vi "Machine job id Read.vi"(11 "Machin ID":string="YSD") -> (0 "error out":errorcluster)   [LabVIEW 2015]
uses:
  Machine id selection.ctl
  PartSetup/Control 1.ctl
  <vilib>/addons/database/NI_Database_API.lvlib
  <vilib>/addons/database/Connection.llb/DB Tools Open Connec (String).vi
  <vilib>/addons/database/_DB Variant To Data/Database Variant To Data.xnode
  Galobal variable_TI.vi
panel:
  out "error out 2":errorcluster
  out "appended array":string[](array[string])
  out "Array 3":string[][](array[string])
  out "element":cluster{"Array":string[][]}
  out "data":string[][](array[string])
  out "Array 2":T1[](array[typedef])
  in  "Enum":T2
  out "Array":cluster{"Array":string[][]}[](array[cluster])
  in  "Cluster":cluster{"Array":string[][]}
  # "First motor testing Parameter"
  # "Printing Info"
  # "Second motor testing Parameter"
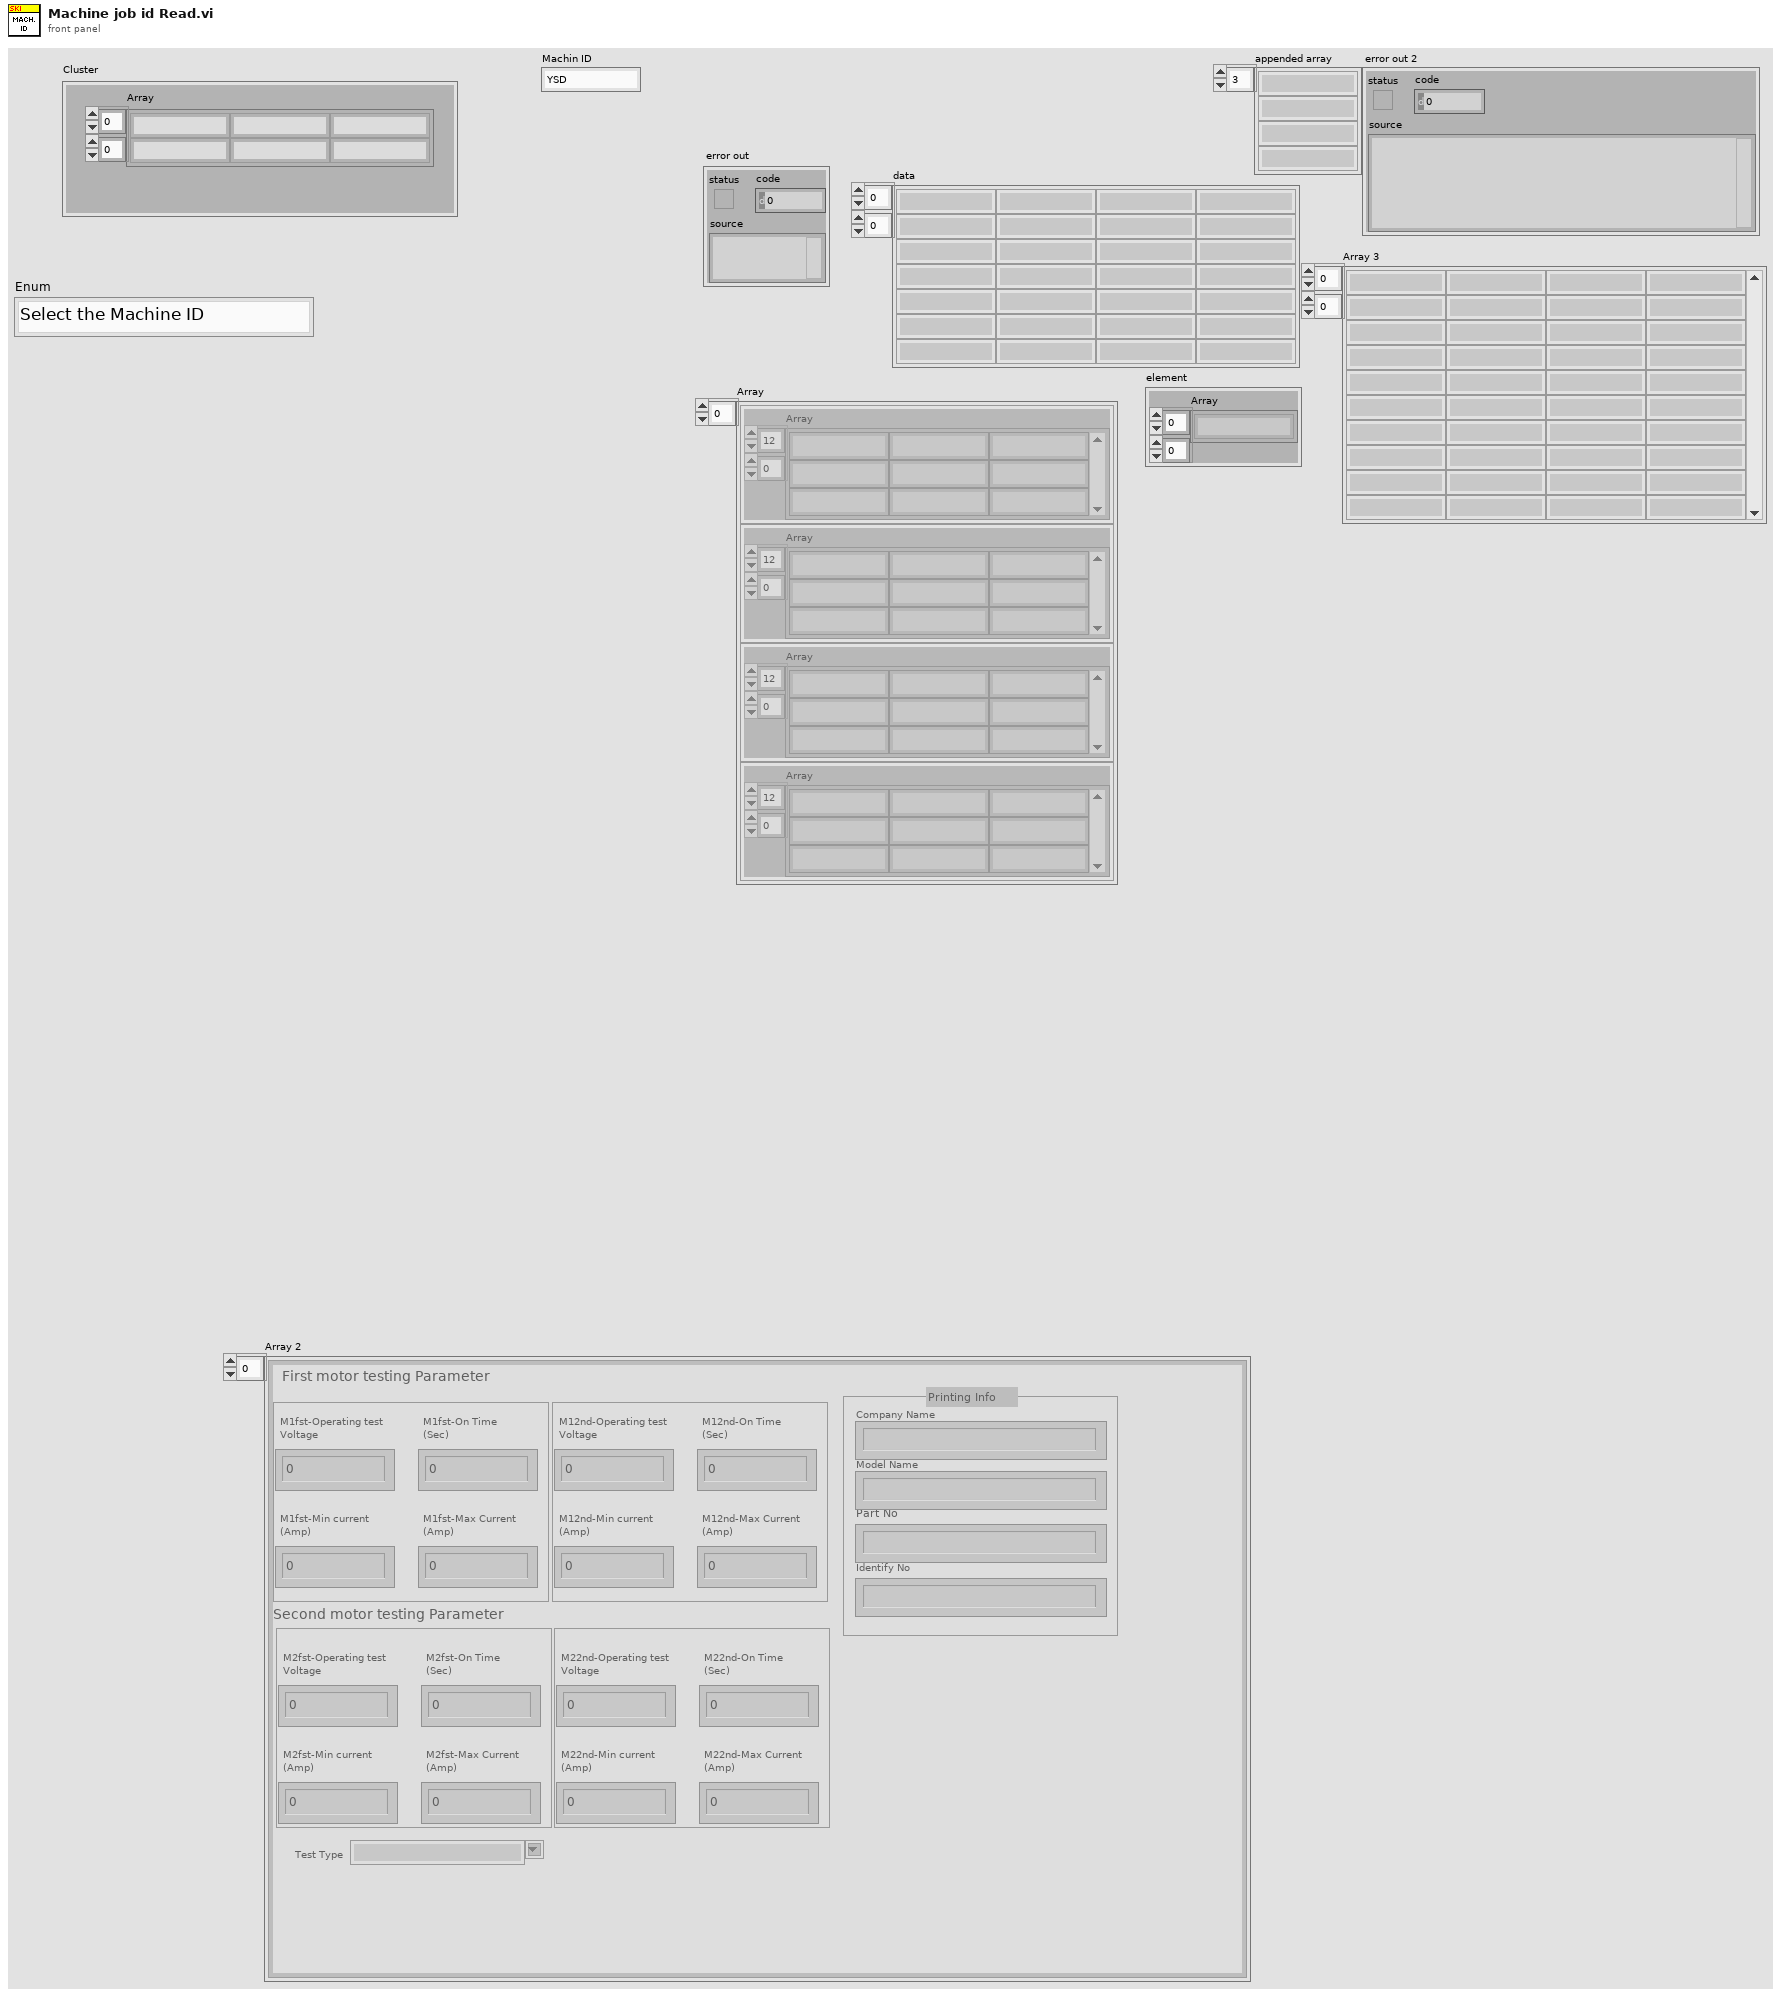
[diagram p1: front panel]
types:
  T1 = typedef "Control 1.ctl" = cluster{"Model Name":string, "Company Name":string, "Part No":string, "Identify No":string, "M1fst-Operating test\nVoltage":dbl, "M1fst-On Time \n(Sec)":dbl, "M1fst-Min current \n(Amp)":dbl, "M1fst-Max Current\n(Amp)":dbl, "M12nd-Operating test\nVoltage":dbl, "M12nd-On Time \n(Sec)":dbl, "M12nd-Min current \n(Amp)":dbl, "M12nd-Max Current\n(Amp)":dbl, "M2fst-Operating test\nVoltage":dbl, "M2fst-On Time \n(Sec)":dbl, "M2fst-Min current \n(Amp)":dbl, "M2fst-Max Current\n(Amp)":dbl, "M22nd-Operating test\nVoltage":dbl, "M22nd-On Time \n(Sec)":dbl, "M22nd-Min current \n(Amp)":dbl, "M22nd-Max Current\n(Amp)":dbl, "Test Type ":string}
  T2 = typedef "Machine id selection.ctl" = enum16{"Select the Machine ID", "YCA", "YHB", "YSD", "Job_Id-62"}
  T3 = typedef "NI_Database_API.lvlib/Conn ObjectReference.ctl" = refnum<k1>
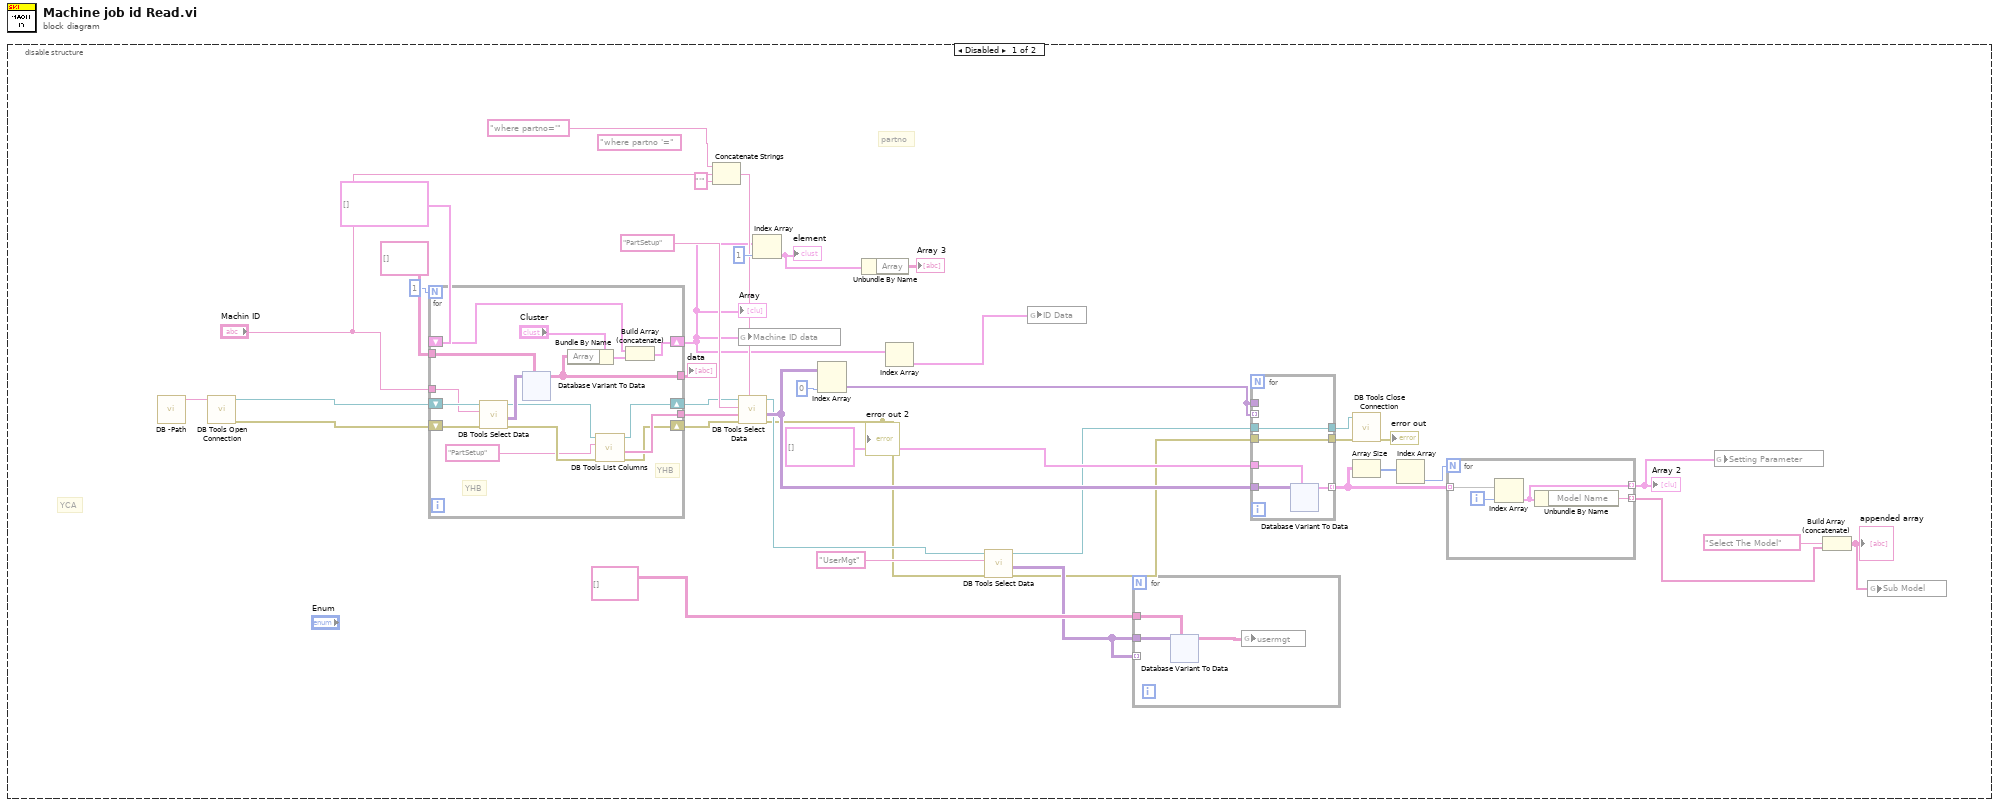
[diagram p0: block diagram]
diagram:
  n1 = disable-structure shown="Disabled" {
    frame Disabled {
      (unwired) "where partno '=" ("condition")
      # "partno"
      # "YCA"
      n2 = call "DB -Path.vi"() -> ("String"=w41:string)  [unwired: 11 in]
      n3 = call-poly <vilib>:"DB Tools Open Connection.vi"("connection information"=w41) -> ("error out"=w19:errorcluster, "connection reference"=w20:T3)  [unwired: 7 in]
      n4 = for {
        N: 1 -> [_]
        shift-right: [w762] -> w35
        shift-left: w20 -> [w774]
        shift-right: [w760] -> w33
        shift-left: w19 -> [w773]
        tunnel: string[][] [] -> [w771]
        shift-right: [w768] -> w2
        shift-left: cluster{"Array":string[][]}[] [] -> [w767]
        tunnel: [w766] -> w24
        tunnel: "Machin ID" -> [w764]
        tunnel: [w765] -> w5
        # "YHB"
        # "YHB"
        n5 = call <vilib>:"DB Tools Select Data.vi"("error in (no error)"=w773, "table"=w764, "connection reference"=w774) -> ("error out"=w761:errorcluster, "data"=w772:variant[][], "connection reference out"=w763:T3)  [unwired: 3 in]
        n6 = xnode "Database Variant To Data"("database variant"=w772, "type"=w771) -> ("data"=w766:string[][])  [unwired: 1 in, 1 out]
        n7 = Bundle By Name(cluster="Cluster", "Array"=w766) -> (w769:cluster{"Array":string[][]})
        n8 = call <vilib>:"DB Tools List Columns.vi"("error in (no error)"=w761, "table"="PartSetup", "connection reference"=w763) -> ("error out"=w760:errorcluster, "columns"=w765:string[], "connection reference out"=w762:T3)  [unwired: 1 in, 1 out]
        n9 = Build Array (concatenate)(w767, w769) -> (w768:cluster{"Array":string[][]}[])
      }
      "Array" <- w2
      "data" <- w24
      n10 = Concatenate Strings("where partno='" ("condition"), "Machin ID", "'" ("string")) -> (w6:string)
      n11 = global write "Galobal variable_TI.vi" "Machine ID data"(w2) -> ()
      n12 = call <vilib>:"DB Tools Select Data.vi"("condition"=w6, "error in (no error)"=w33, "columns"=w5, "table"="PartSetup", "connection reference"=w35) -> ("error out"=w11:errorcluster, "data"=w30:variant[][], "connection reference out"=w16:T3)  [unwired: 1 in]
      "error out 2" <- w11
      n13 = Index Array(array=w2, index=1) -> (element=w22:cluster{"Array":string[][]})
      "element" <- w22
      n14 = Index Array(array=w30, index (col)=0 ("disabled index (col)")) -> (element=w31:variant[])  [unwired: 1 in]
      n15 = Unbundle By Name(w22) -> ("Array"=→"Array 3":string[][])
      n16 = Index Array(array=w2) -> (element=w1:cluster{"Array":string[][]})  [unwired: 1 in]
      n17 = call <vilib>:"DB Tools Select Data.vi"("error in (no error)"=w11, "table"="UserMgt", "connection reference"=w16) -> ("error out"=w10:errorcluster, "data"=w12:variant[][], "connection reference out"=w15:T3)  [unwired: 3 in]
      n18 = global write "Galobal variable_TI.vi" "ID Data"(w1) -> ()
      n19 = for {
        tunnel: string[][] [] -> [w44]
        tunnel: w12 -> [w43]
        tunnel: w12 -> [_] mode=indexing
        n20 = xnode "Database Variant To Data"("database variant"=w43, "type"=w44) -> ("data"=w42:string[][])  [unwired: 1 in, 1 out]
        n21 = global write "Galobal variable_TI.vi" "usermgt"(w42) -> ()
      }
      n22 = for {
        tunnel: w15 -> [w97]
        tunnel: w10 -> [w96]
        tunnel: w31 -> [_]
        tunnel: [w97] -> w34
        tunnel: [w96] -> w32
        tunnel: w31 -> [_] mode=indexing
        tunnel: w30 -> [w94]
        tunnel: T1[] [] -> [w95]
        tunnel: [w93] -> w26 mode=indexing
        n23 = xnode "Database Variant To Data"("database variant"=w94, "type"=w95) -> ("data"=w93:T1[])  [unwired: 1 in, 1 out]
      }
      n24 = call <vilib>:"DB Tools Close Connection.vi"("error in (no error)"=w32, "connection reference"=w34) -> ("error out"=→"error out":errorcluster)  [unwired: 5 in]
      n25 = Array Size(array=w26) -> (size(s)=w28:i32[])
      n26 = Index Array(array=w28) -> (element=w27:i32)  [unwired: 1 in]
      n27 = for {
        N: w27 -> [_]
        tunnel: w26 -> [w91] mode=indexing
        tunnel: [w90] -> w25 mode=indexing
        tunnel: [w89] -> w18 mode=indexing
        i -> [w92]
        n28 = Index Array(array=w91, index=w92) -> (element=w90:T1)
        n29 = Unbundle By Name(w90) -> ("Model Name"=w89:string)
      }
      "Array 2" <- w25
      n30 = global write "Galobal variable_TI.vi" "Setting Parameter"(w25) -> ()
      n31 = Build Array (concatenate)("Select The Model", w18) -> (w3:string[])
      "appended array" <- w3
      n32 = global write "Galobal variable_TI.vi" "Sub Model"(w3) -> ()
    }
    frame Enabled {
    }
  }
